vi "Control Mode Read Array.vi"(8 "error in":errorcluster, 11 "Cycler in":refnum<class "Cycler.lvclass">) -> (0 "error out":errorcluster, 1 "Changed or First Call?":bool, 2 "Control Mode CTL":u16[](array[numeric]), 3 "Cycler out":refnum<class "Cycler.lvclass">)   [LabVIEW 2023, in "Cycler.lvclass"]
uses:
  Cycler.lvclass
  Cycler.lvclass/Cycler.ctl
  Low Level Capabilities/Control Mode/Control Mode.lvclass
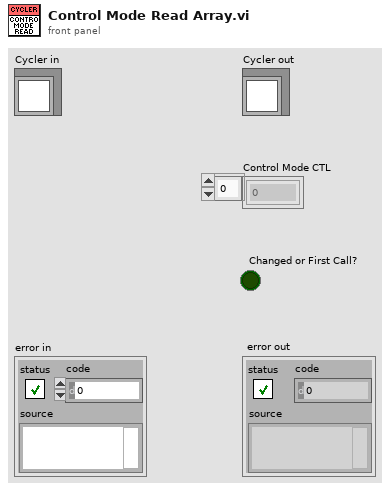
[diagram p1: front panel]
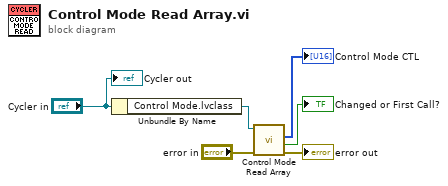
[diagram p0: block diagram]
diagram:
  n1 = Unbundle By Name("Cycler in") -> ("Control Mode.lvclass"=w4:refnum<class "Control Mode.lvclass">)
  n2 = call-dynamic "Control Mode Read Array.vi"("error in"="error in", "Control Mode in"=w4) -> ("error out"=→"error out":errorcluster, "Changed or First Call?"=→"Changed or First Call?":bool, "Control Mode CTL"=→"Control Mode CTL":u16[])  [unwired: 6 in, 1 out]
  "Cycler out" <- "Cycler in"
